vi "Feeder Lift.vi"(8 "error in (no error)":errorcluster) -> (0 "error out":errorcluster)   [LabVIEW 2014]
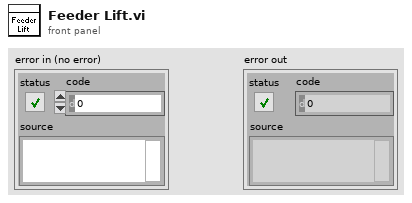
[diagram p1: front panel]
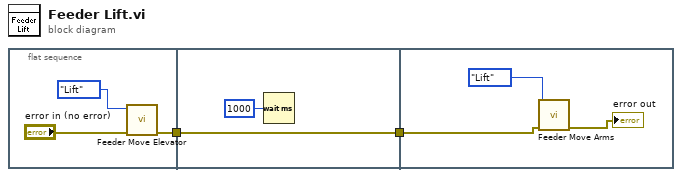
[diagram p0: block diagram]
diagram:
  n1 = flat-sequence {
    tunnel: [w3] -> w1
    tunnel: [w6] -> w2
    tunnel: w1 -> [w6]
    tunnel: w2 -> [w9]
    frame #0 {
      n2 = call "Feeder Move Elevator.vi"("error in (no error)"="error in (no error)", "Action"=enum16{"Drop", "Lift"}."Lift") -> ("error out"=w3:errorcluster)  [unwired: 9 in]
    }
    frame #1 {
      n3 = Wait (ms)(milliseconds to wait=u32 1000) -> ()  [unwired: 1 out]
    }
    frame #2 {
      n4 = call "Feeder Move Arms.vi"("error in (no error)"=w9, "Action"=enum16{"Drop", "Lift"}."Lift") -> ("error out"=→"error out":errorcluster)  [unwired: 9 in]
    }
  }
